vi "Bridge_Readback.vi"(0 "HSDIO Sessions":T4, 2 "USID":T3 max=15, 5 "Error In":errorcluster, 8 "Reg_Address_to_Read":T1={"First Reg Address"=31, "Num of Reg to Read"=31} {"Num of Reg to Read" min=1; "First Reg Address" format="%.0x"}, 9 "Bit_Location(LSB)":u8 max=7, 11 "#ofBits":u8=4 min=1 max=8) -> (14 "Registers_Readback":i32[](array[numeric]), 16 "Data_Readback":u8[](array[numeric])=[31, 144, 7], 17 "Waveform Graph":digitalwaveform(graph), 18 "Converted Data":T2 {"Register" max=31 format="%.0x"; "Slave Address" max=15 format="%.0x"}, 19 "Error Out":errorcluster)   [LabVIEW 2013]
uses:
  Controls/USID.ctl
  Controls/Reg_Address_Data.ctl
panel:
  out "Value":u8=184
  # "Specific Bits to read"
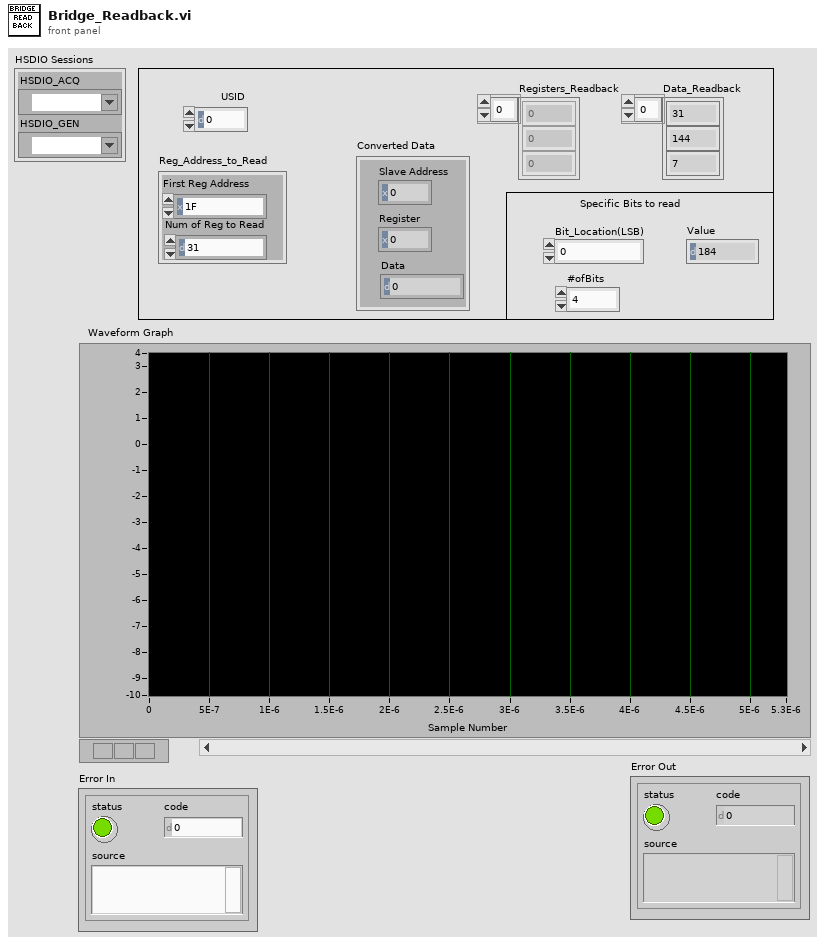
[diagram p1: front panel]
types:
  T1 = cluster{"First Reg Address":u8, "Num of Reg to Read":u8}
  T2 = cluster{"Slave Address":u8, "Register":u8, "Data":u8}
  T3 = typedef "USID.ctl" = u8
  T4 = cluster{"HSDIO_ACQ":refnum<k15>, "HSDIO_GEN":refnum<k15>}
  T5 = typedef "Reg_Address_Data.ctl" = cluster{"Address":u8, "Data":u8}
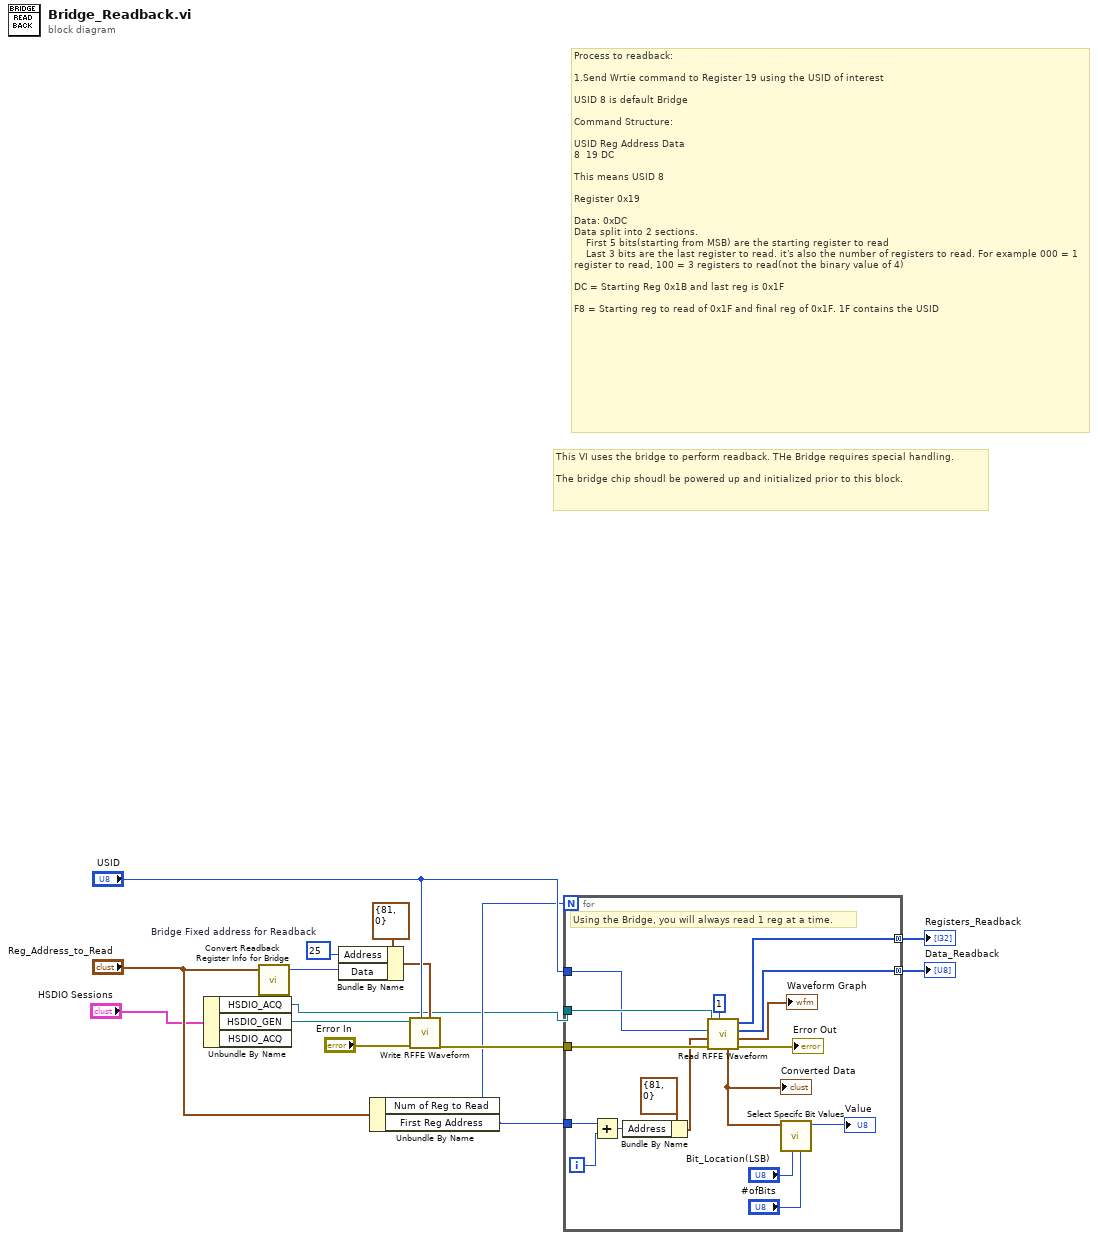
[diagram p0: block diagram]
diagram:
  w11 = u8 25  # Bridge Fixed address for Readback
  # "Process to readback:\n\n1.Send Wrtie command to Register 19 using the USID of interest\n\nUSID 8 is default Bridge\n\nCommand Structure:\n\nUSID Reg Address Data\n8  19 DC\n\nThis means USID 8\n\nRegister 0x19\n\nData: 0xDC\nData split into 2 sections. \n    First 5 bits(starting from MSB) are the starting register to read\n    Last 3 bits are the last register to read. it's also the number of registers to read. For example 000 = 1 register to read, 100 = 3 registers to read(not the binary value of 4)\n\nDC = Starting Reg 0x1B and last reg is 0x1F\n\nF8 = Starting reg to read of 0x1F and final reg of 0x1F. 1F contains the USID"
  # "This VI uses the bridge to perform readback. THe Bridge requires special handling.\n\nThe bridge chip shoudl be powered up and initialized prior to this block."
  n1 = Unbundle By Name("HSDIO Sessions") -> ("HSDIO_ACQ"=w1:refnum<k15>, "HSDIO_GEN"=w2:refnum<k15>)  [unwired: 1 out]
  n2 = call "Convert Readback Register Info for Bridge.vi"("Reg_Address_to_Read"="Reg_Address_to_Read") -> ("number"=w4:u32)  [unwired: 4 in]
  n3 = Bundle By Name(cluster=T5 {"Address"=81, "Data"=0} ("Reg_Address_Data"), "Address"=w11, "Data"=w4) -> (w10:T5)
  n4 = Unbundle By Name("Reg_Address_to_Read") -> ("Num of Reg to Read"=w6:u8, "First Reg Address"=w9:u8)
  n5 = call "Write RFFE Waveform.vi"("Reg_Address_Data"=w10, "USID"="USID", "error in (no error)"="Error In", "instrument handle"=w2) -> ("error out"=w15:errorcluster)  [unwired: 5 in, 2 out]
  n6 = for {
    N: w6 -> [_]
    tunnel: w15 -> [w32]
    tunnel: w1 -> [w31]
    tunnel: "USID" -> [w29]
    tunnel: w9 -> [w22]
    tunnel: [w19] -> w8 mode=concatenating
    tunnel: [w18] -> w7 mode=concatenating
    i -> [w21]
    # "Using the Bridge, you will always read 1 reg at a time."
    n7 = Add(x=w22, y=w21) -> (x+y=w20:i32)
    n8 = Bundle By Name(cluster=T5 {"Address"=81, "Data"=0} ("Reg_Address_Data"), "Address"=w20) -> (w23:T5)
    n9 = call "Read RFFE Waveform.vi"("Number of Registers to Read"=u8 1, "error in (no error)"=w32, "Reg_Address_Data"=w23, "USID"=w29, "HSDIO_VISA"=w31) -> ("error out"=→"Error Out":errorcluster, "Waveform Graph"=→"Waveform Graph":digitalwaveform, "Ext_Read_Data"=w18:u8[], "Ext_Read_Reg"=w19:i32[], "Converted Data"=w27:T2)  [unwired: 2 in]
    "Converted Data" <- w27
    n10 = call "Select Specifc Bit Values.vi"("#ofBits"="#ofBits", "Bit_Location(LSB)"="Bit_Location(LSB)", "Converted Data"=w27) -> ("Bits"=→"Value":u8)  [unwired: 8 in]
  }
  "Registers_Readback" <- w8
  "Data_Readback" <- w7
